vi "Populate OD.vi"(8 "error in":errorcluster, 10 "EDS":refnum<class "Electronic Datasheet.lvclass">, 11 "Object Dictionary UI in":refnum<class "Object Dictionary UI.lvclass">) -> (0 "error out":errorcluster, 3 "Object Dictionary UI out":refnum<class "Object Dictionary UI.lvclass">)   [LabVIEW 2020, in "Object Dictionary UI.lvlib" / "Object Dictionary UI.lvclass"]
uses:
  Object Dictionary UI.lvclass
  Object Dictionary UI.lvclass/Object Dictionary UI.ctl
  EDS-File-Viewer/source/Electronic Datasheet/Electronic Datasheet.lvclass
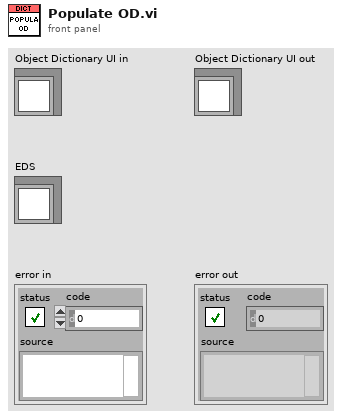
[diagram p1: front panel]
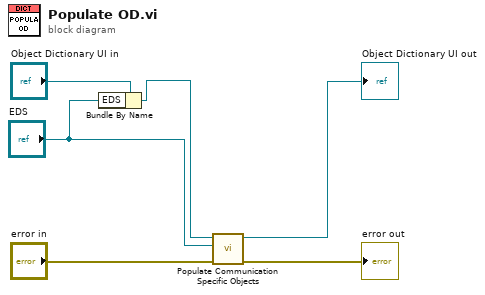
[diagram p0: block diagram]
diagram:
  n1 = Bundle By Name(cluster="Object Dictionary UI in", "EDS"="EDS") -> (w2:refnum<class "Object Dictionary UI.lvclass">)
  n2 = call "Populate Communication Specific Objects.vi"("error in"="error in", "EDS"="EDS", "object in"=w2) -> ("error out"=→"error out":errorcluster, "object out"=→"Object Dictionary UI out":refnum<class "Object Dictionary UI.lvclass">)  [unwired: 7 in]
